vi "svx_DAQ_ClockRateFromFrequency.vi"(8 "error in (no error)":errorcluster, 10 "Max Frequency of Interest":dbl, 11 "Device Max Sample Rate":dbl=inf) -> (0 "error out":errorcluster, 2 "Sample Clock Rate":dbl)   [LabVIEW 2017, in "SVX NI-DAQmx AI Configuration XControl.xctl"]
uses:
  <vilib>/addons/Sound and Vibration/svt_DAQmx/Configuration XControl/SVX NI-DAQmx AI Configuration XControl.xctl
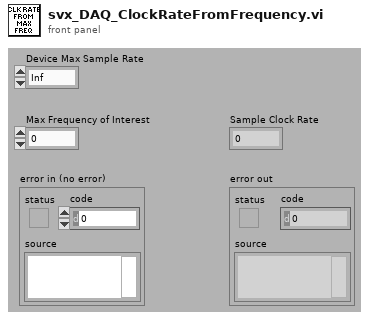
[diagram p1: front panel]
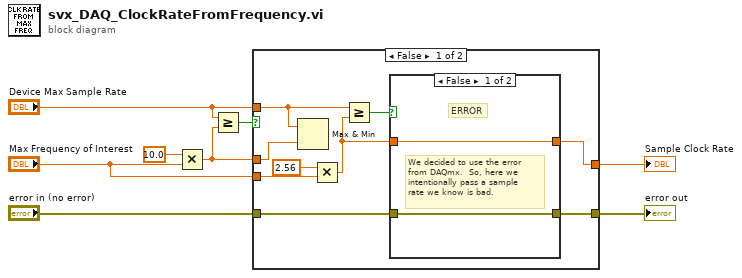
[diagram p0: block diagram]
diagram:
  n1 = Multiply(x=10.0, y="Max Frequency of Interest") -> (x*y=w5:dbl)
  n2 = Greater Or Equal?(x="Device Max Sample Rate", y=w5) -> (x >= y?=w4:bool)
  n3 = case shown="False" w4 {
    tunnel: [w9 w23] -> w7
    tunnel: w5 -> [w11 w23]
    tunnel: "Max Frequency of Interest" -> [w17 _]
    tunnel: "Device Max Sample Rate" -> [w12 _]
    tunnel: [w15 w22] -> w2
    tunnel: "error in (no error)" -> [w14 w22]
    frame False {
      n4 = Max & Min(x=w12, y=w11) -> ()  [unwired: 2 out]
      n5 = Multiply(x=2.56, y=w17) -> (x*y=w10:dbl)
      n6 = Greater Or Equal?(x=w12, y=w10) -> (x >= y?=w16:bool)
      n7 = case shown="False" w16 {
        tunnel: [w19 w21] -> w15
        tunnel: w14 -> [w19 w21]
        tunnel: [w18 w20] -> w9
        tunnel: w10 -> [w18 w20]
        frame False {
          # "We decided to use the error\nfrom DAQmx.  So, here we\nintentionally pass a sample\nrate we know is bad."
          # "ERROR"
        }
        frame True {
        }
      }
    }
    frame True {
    }
  }
  "Sample Clock Rate" <- w7
  "error out" <- w2
